vi "Remove Empty Chars.vi"(11 "String with \\00":string) -> (3 "String without \\00":string)   [LabVIEW 2017]
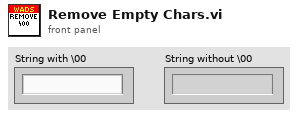
[diagram p1: front panel]
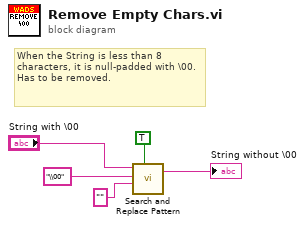
[diagram p0: block diagram]
diagram:
  # "When the String is less than 8 characters, it is null-padded with \\00. Has to be removed."
  n1 = call <vilib>:"Search and Replace Pattern.vi"("string"="String with \\00", "regular expression (\"\")"="\\00" ("regular expression (\"\")"), "replace string (\"\")"="", "replace all? (F)"=TRUE) -> ("result string"=→"String without \\00":string)  [unwired: 1 in, 1 out]
